vi "Parse NMEA String.vi"(11 "NMEA String":string) -> (0 "Error Out":errorcluster, 3 "GPS Data Out":T1 {"Time"."GPS Time of Week" format="%.3f"; "Velocity, Correction & SET"."Extended Navigation Mode" items=["Non Differential"=0, "Code (RTCM Type 1 & 9)"=1, "Code, Single Frequency (WAAS)"=2, "Code, Dual Frequency (WAAS)"=3, "Code, Single Frequency (WCT)"=4, "Code/RCP, Dual Frequency (WCT)"=5, "Code, Single Frequency (RTG)"=6, "Code (RTCM Type 1 & 9) Dual Frequency"=10, "Code/RCP, Dual Frequency (RTG)"=11, "Code, Single Frequency (NCT-RTK)"=12, "Code, Single Frequency (RTCM 18 & 19)"=13, "Code, Single Frequency (RTCM 21 & 22)"=14, "Code, Single Frequency (CMR)"=15, "Code, Dual Frequency (NCT-RTK)"=16, "Code, Dual Frequency (RTCM 18 & 19)"=17, "Code, Dual Frequency (RTCM 20 & 21)"=18, "Code, Dual Frequency (CMR)"=19, "RTK (NCT-RTK)"=20, "RTK (RTCM 18 & 19)"=21, "RTK (RTCM 20 & 21)"=22, "RTK (CMR)"=23, "Code, Single Frequency with SET (RTG)"=24, "Code/RCP, Dual Frequency with SET (RTG)"=25, "RTK Extend"=26]})   [LabVIEW 2011]
panel:
  in  "GPS Data":T1 {"Time"."GPS Time of Week" format="%.3f"; "Velocity, Correction & SET"."Extended Navigation Mode" items=["Non Differential"=0, "Code (RTCM Type 1 & 9)"=1, "Code, Single Frequency (WAAS)"=2, "Code, Dual Frequency (WAAS)"=3, "Code, Single Frequency (WCT)"=4, "Code/RCP, Dual Frequency (WCT)"=5, "Code, Single Frequency (RTG)"=6, "Code (RTCM Type 1 & 9) Dual Frequency"=10, "Code/RCP, Dual Frequency (RTG)"=11, "Code, Single Frequency (NCT-RTK)"=12, "Code, Single Frequency (RTCM 18 & 19)"=13, "Code, Single Frequency (RTCM 21 & 22)"=14, "Code, Single Frequency (CMR)"=15, "Code, Dual Frequency (NCT-RTK)"=16, "Code, Dual Frequency (RTCM 18 & 19)"=17, "Code, Dual Frequency (RTCM 20 & 21)"=18, "Code, Dual Frequency (CMR)"=19, "RTK (NCT-RTK)"=20, "RTK (RTCM 18 & 19)"=21, "RTK (RTCM 20 & 21)"=22, "RTK (CMR)"=23, "Code, Single Frequency with SET (RTG)"=24, "Code/RCP, Dual Frequency with SET (RTG)"=25, "RTK Extend"=26]}
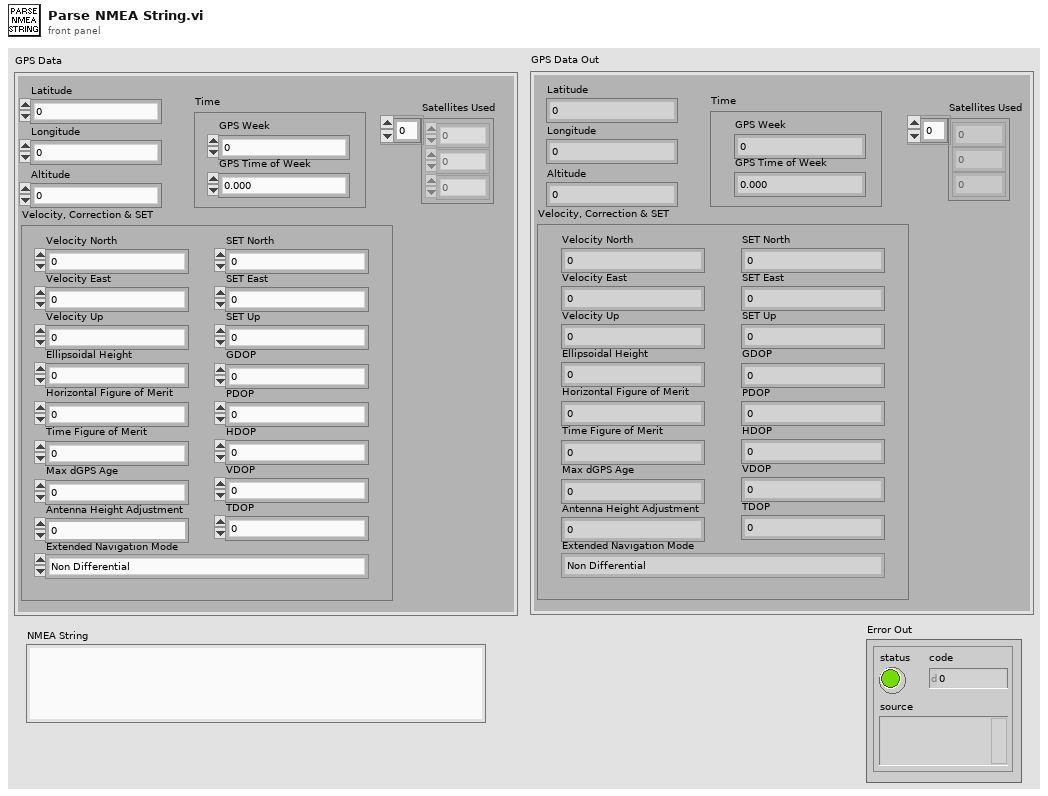
[diagram p1: front panel]
types:
  T1 = cluster{"Latitude":dbl, "Longitude":dbl, "Altitude":dbl, "Velocity, Correction & SET":cluster{"Velocity North":dbl, "Velocity East":dbl, "Velocity Up":dbl, "Ellipsoidal Height":dbl, "GDOP":sgl, "PDOP":sgl, "HDOP":sgl, "VDOP":sgl, "TDOP":sgl, "Horizontal Figure of Merit":u8, "Time Figure of Merit":u8, "Max dGPS Age":sgl, "Extended Navigation Mode":u8, "Antenna Height Adjustment ":dbl, "SET North":i32, "SET East":i32, "SET Up":i32}, "Time":cluster{"GPS Week":u16, "GPS Time of Week":sgl}, "Satellites Used":i32[]}
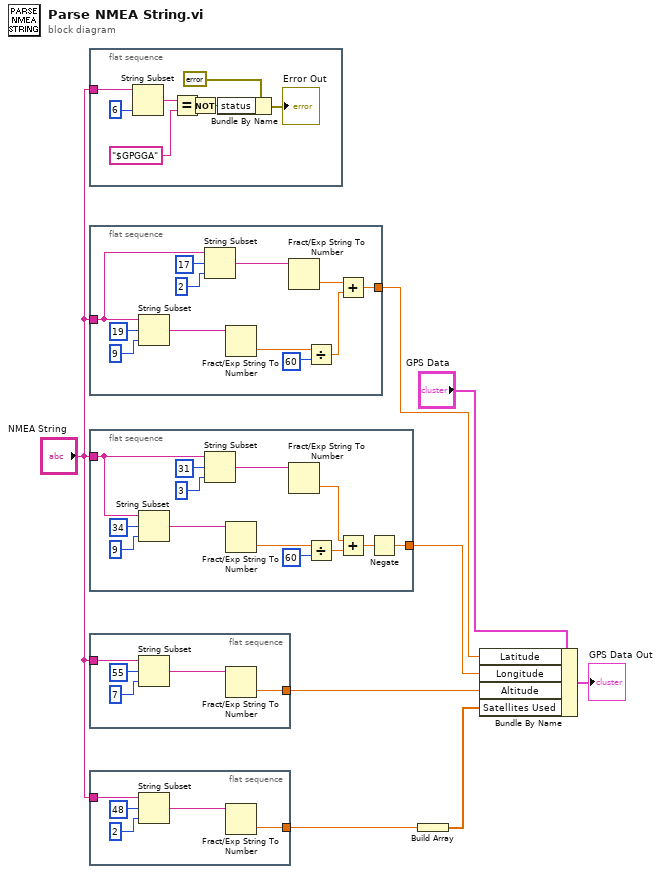
[diagram p0: block diagram]
diagram:
  n1 = flat-sequence {
    tunnel: "NMEA String" -> [w13]
    frame #0 {
      n2 = String Subset(string=w13, length (rest)=6 ("length (rest)")) -> (substring=w15:string)  [unwired: 1 in]
      n3 = Equal?(x=w15, y="$GPGGA") -> (x = y?=w10:bool)
      n4 = Not(x=w10) -> (.not. x?=w9:bool)
      n5 = Bundle By Name(cluster=errorcluster {"status"=FALSE, "code"=0, "source"=""} ("error constant"), "status"=w9) -> (→"Error Out":errorcluster)
    }
  }
  n6 = flat-sequence {
    tunnel: "NMEA String" -> [w18]
    tunnel: [w17] -> w6
    frame #0 {
      n7 = String Subset(string=w18, offset (0)=19, length (rest)=9 ("length (rest)")) -> (substring=w24:string)
      n8 = String Subset(string=w18, offset (0)=17, length (rest)=2 ("length (rest)")) -> (substring=w23:string)
      n9 = Fract/Exp String To Number(string=w24) -> (number=w26:dbl)  [unwired: 3 in, 1 out]
      n10 = Fract/Exp String To Number(string=w23) -> (number=w28:dbl)  [unwired: 3 in, 1 out]
      n11 = Divide(x=w26, y=60) -> (x/y=w27:dbl)
      n12 = Add(x=w28, y=w27) -> (x+y=w17:dbl)
    }
  }
  n13 = flat-sequence {
    tunnel: "NMEA String" -> [w30]
    tunnel: [w29] -> w5
    frame #0 {
      n14 = String Subset(string=w30, offset (0)=34, length (rest)=9 ("length (rest)")) -> (substring=w41:string)
      n15 = String Subset(string=w30, offset (0)=31, length (rest)=3 ("length (rest)")) -> (substring=w36:string)
      n16 = Fract/Exp String To Number(string=w41) -> (number=w37:dbl)  [unwired: 3 in, 1 out]
      n17 = Fract/Exp String To Number(string=w36) -> (number=w39:dbl)  [unwired: 3 in, 1 out]
      n18 = Divide(x=w37, y=60) -> (x/y=w40:dbl)
      n19 = Add(x=w39, y=w40) -> (x+y=w31:dbl)
      n20 = Negate(x=w31) -> (-x=w29:dbl)
    }
  }
  n21 = flat-sequence {
    tunnel: "NMEA String" -> [w43]
    tunnel: [w42] -> w4
    frame #0 {
      n22 = String Subset(string=w43, offset (0)=55, length (rest)=7 ("length (rest)")) -> (substring=w44:string)
      n23 = Fract/Exp String To Number(string=w44) -> (number=w42:dbl)  [unwired: 3 in, 1 out]
    }
  }
  n24 = flat-sequence {
    tunnel: "NMEA String" -> [w48]
    tunnel: [w47] -> w2
    frame #0 {
      n25 = String Subset(string=w48, offset (0)=48, length (rest)=2 ("length (rest)")) -> (substring=w51:string)
      n26 = Fract/Exp String To Number(string=w51) -> (number=w47:dbl)  [unwired: 3 in, 1 out]
    }
  }
  n27 = Build Array(w2) -> (w3:dbl[])
  n28 = Bundle By Name(cluster="GPS Data", "Latitude"=w6, "Longitude"=w5, "Altitude"=w4, "Satellites Used"=w3) -> (→"GPS Data Out":T1)
